vi "chart_vs_graph.vi"() -> ()   [LabVIEW 2021]
panel:
  out "Waveform Graph":dbl[](graph)
  out "Waveform Chart":dbl(graph)
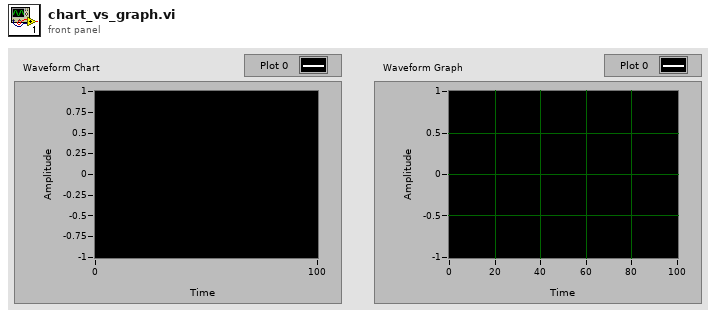
[diagram p1: front panel]
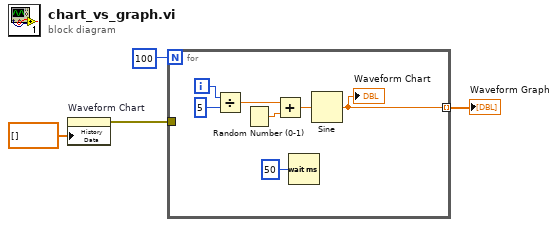
[diagram p0: block diagram]
diagram:
  n1 = property on="Waveform Chart" class="WFChart (strict)"("History Data"=dbl[] []) -> (error out=w1:errorcluster)  [unwired: 2 in, 1 out]
  n2 = for {
    N: 100 -> [_]
    tunnel: [w9] -> w3 mode=indexing
    tunnel: w1 -> [_]
    i -> [w11]
    n3 = Divide(x=w11, y=5) -> (x/y=w7:dbl)
    n4 = Random Number (0-1)() -> (number: 0 to 1=w8:dbl)
    n5 = Add(x=w7, y=w8) -> (x+y=w6:dbl)
    n6 = Wait (ms)(milliseconds to wait=u32 50) -> ()  [unwired: 1 out]
    n7 = Sine(x=w6) -> (sin(x)=w9:dbl)
    "Waveform Chart" <- w9
  }
  "Waveform Graph" <- w3
